vi "UDPSingleCommandSender.vi"(9 "Command":T2, 10 "Tello IP":T1="192.168.1.10") -> (2 "Return":string)   [LabVIEW 2018]
uses:
  Library/Central Controller/TypeDef/TelloCommands.ctl
  Library/Central Controller/TypeDef/TelloIP.ctl
  Library/Simple UDP Message/Simple UDP Message.lvlib
panel:
  out "iteration (ms)":u32
  in  "timeout (ms)":i32=5000
  out "iteration":i32
  in  "Send Cmd":bool
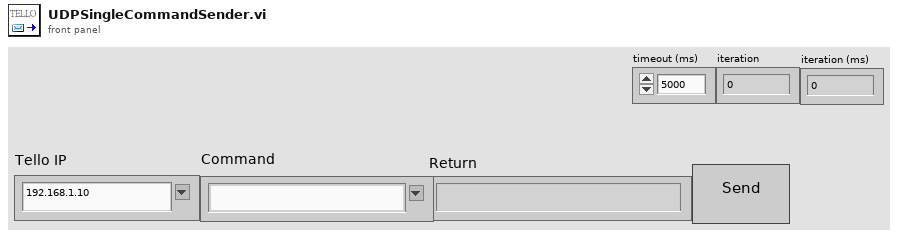
[diagram p1: front panel]
types:
  T1 = typedef "TelloIP.ctl" = string
  T2 = typedef "TelloCommands.ctl" = string
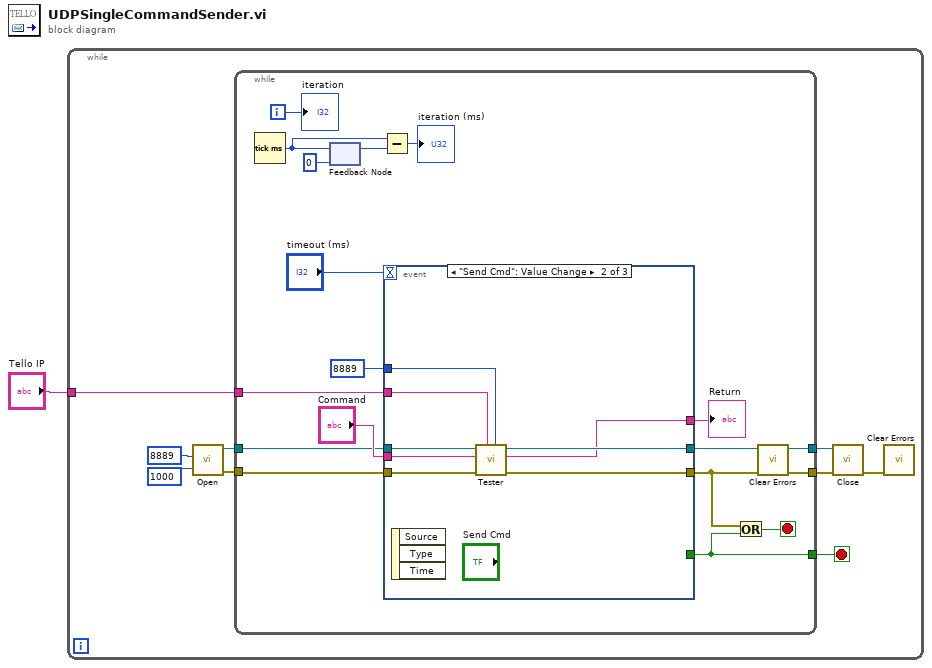
[diagram p0: block diagram]
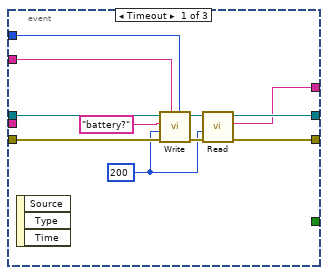
[diagram p2: hidden frame]
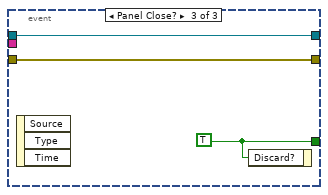
[diagram p3: hidden frame]
diagram:
  n1 = while {
    tunnel: "Tello IP" -> [w9]
    stop <- w10 stop-if-true
    n2 = call "Open.vi"("timeout ms (60000)"=1000 ("timeout ms (25000)"), "port"=u16 8889) -> ("error out"=w8:errorcluster, "connection ID"=w7:refnum<k16>)  [unwired: 8 in]
    n3 = while {
      tunnel: [w22] -> w10
      tunnel: w9 -> [w24]
      tunnel: w8 -> [w15]
      tunnel: w7 -> [w14]
      tunnel: [w13] -> w6
      tunnel: [w12] -> w5
      i -> [w20]
      stop <- w23 stop-if-true
      n4 = Tick Count (ms)() -> (millisecond timer value=w19:u32)
      n5 = feedback-in #1(w19) -> ()
      n6 = feedback #1(u32 0 ("millisecond timer value")) -> (w18:u32)
      n7 = Subtract(x=w19, y=w18) -> (x-y=→"iteration (ms)":u32)
      n8 = event shown="[1] \"Send Cmd\": Value Change" {
        selector: _ -> [_ _ _]
        dyn-events: _ -> [_ _ _]
        timeout: "timeout (ms)" -> [_ _ _]
        tunnel: w14 -> [w38 w44 w48]
        tunnel: u16 8889 ("port or service name") -> [w28 w40 _]
        tunnel: w15 -> [w37 w43 w47]
        tunnel: [w33 w46 w47] -> w11
        tunnel: [w31 w45 w48] -> w12
        tunnel: "Command" -> [_ w39 _]
        tunnel: [w30 w41 _] -> w26
        tunnel: [_ _ w49] -> w22
        tunnel: w24 -> [w35 w42 _]
        event Timeout {
          w29 = 200 ("timeout ms (25000)")
          n9 = event-data() -> ()  [unwired: 1 in, 3 out]
          n10 = call "Write.vi"("port or service name"=w28, "IP"=w35, "error in (no error)"=w37, "timeout ms (25000)"=w29, "data in"="battery?", "connection ID"=w38) -> ("error out"=w34:errorcluster, "connection ID"=w32:refnum<k16>)  [unwired: 4 in]
          n11 = call "Read.vi"("error in (no error)"=w34, "timeout ms (25000)"=w29, "connection ID"=w32) -> ("error out"=w33:errorcluster, "data out"=w30:string, "connection ID"=w31:refnum<k16>)  [unwired: 4 in, 2 out]
        }
        event "Send Cmd": Value Change {
          n12 = event-data() -> ()  [unwired: 1 in, 3 out]
          n13 = call "Tester.vi"("port or service name"=w40, "IP"=w42, "error in (no error)"=w43, "Command"=w39, "connection ID"=w44) -> ("error out"=w46:errorcluster, "checker"=w41:string, "connection ID"=w45:refnum<k16>)  [unwired: 3 in, 1 out]
        }
        event Panel Close? {
          w49 = TRUE ("Discard?")
          n14 = event-data() -> ()  [unwired: 1 in, 3 out]
          n15 = event-data("Discard?"=w49) -> ()  [unwired: 1 in, 1 out]
        }
      }
      "Return" <- w26
      n16 = Or(x=w11, y=w22) -> (x .or. y?=w23:bool)
      n17 = call <vilib>:"Clear Errors.vi"("error in (no error)"=w11) -> ("error out"=w13:errorcluster)  [unwired: 5 in, 1 out]
      "iteration" <- w20
    }
    n18 = call "Close.vi"("error in (no error)"=w6, "connection ID"=w5) -> ("error out"=w4:errorcluster)  [unwired: 9 in]
    n19 = call <vilib>:"Clear Errors.vi"("error in (no error)"=w4) -> ()  [unwired: 5 in, 2 out]
  }
